vi "process_simple_analysis.vi"(8 "error in (no error)":errorcluster) -> (0 "error out":errorcluster)   [LabVIEW 2010]
uses:
  typedefs/control_analysis_enum.ctl
  typedefs/data_cluster.ctl
panel:
  out "Display sample rate":dbl caption="[Hz]"
  in  "Pixels to integrate":i32=1 min=1 max=1000 step=1
  in  "Display":enum32{"Raw data", "Integrated data"}(radio)
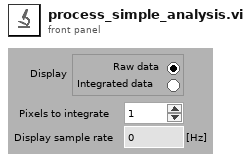
[diagram p1: front panel]
types:
  T1 = typedef "data_cluster.ctl" = cluster{"t0":dbl, "dt":dbl, "Channels":dbl[][]}
  T2 = typedef "control_analysis_enum.ctl" = enum16{"Init", "Analyze", "Reset", "Stop", "Quit"}
  T3 = cluster{"Control Analysis Enum":T2, "variant":variant}
  T4 = cluster{"Data_to_Display_Queue":refnum<queue>, "Data_to_Storage_Queue":refnum<queue>}
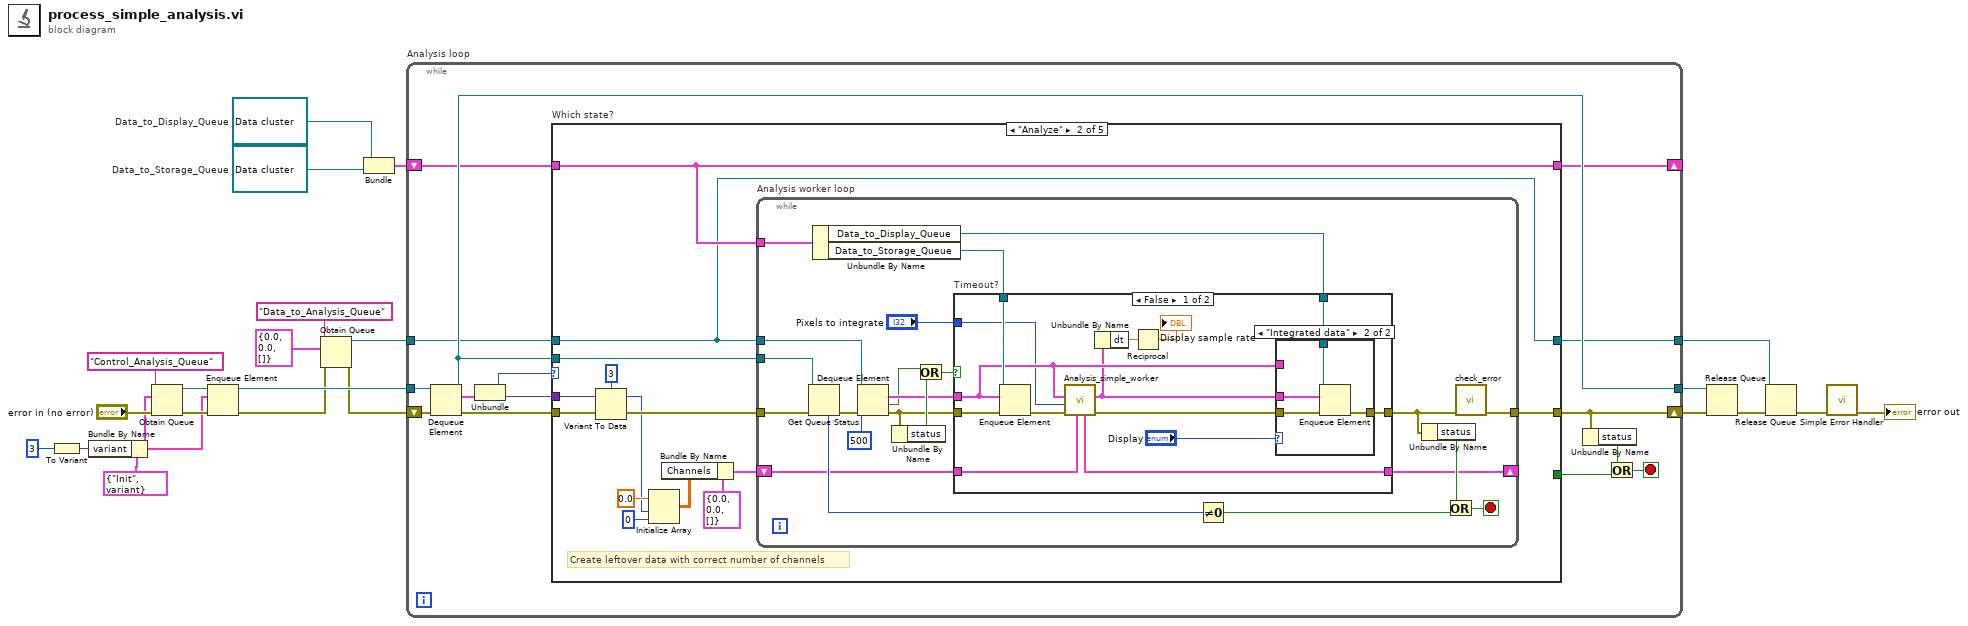
[diagram p0: block diagram]
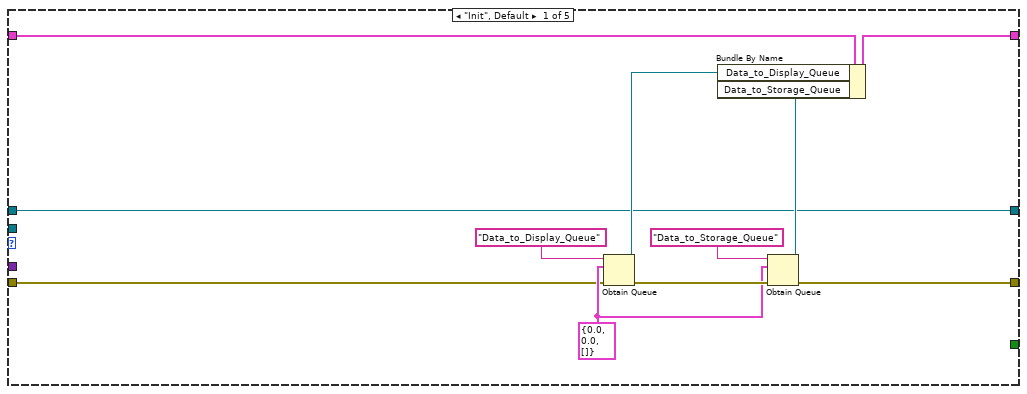
[diagram p2: hidden frame]
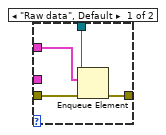
[diagram p3: hidden frame]
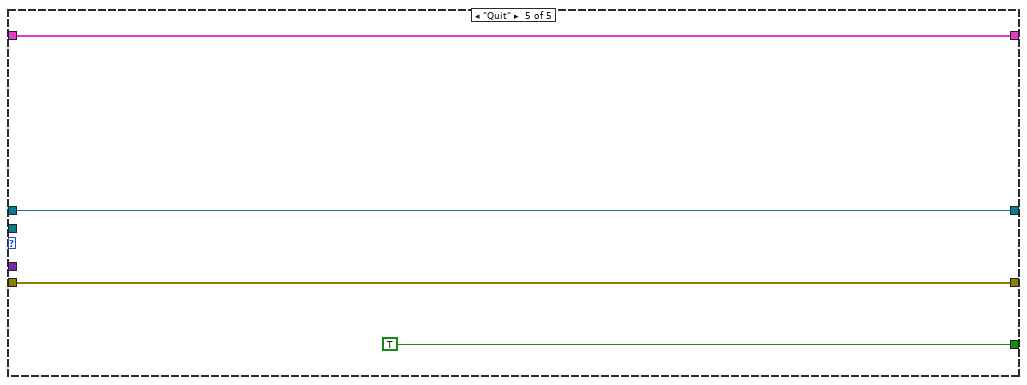
[diagram p7: hidden frame]
diagram:
  w7 = refnum<queue> refnum  # Data_to_Storage_Queue
  w8 = refnum<queue> refnum  # Data_to_Display_Queue
  n1 = To Variant(anything=3) -> (Variant=w2:variant)
  n2 = Bundle By Name(cluster=T3 {"Control Analysis Enum"=enum."Init", "variant"=variant}, "variant"=w2) -> (w1:T3)
  n3 = Obtain Queue(name (unnamed)="Control_Analysis_Queue", element data type=w1, error in (no error)="error in (no error)") -> (queue out=w20:refnum<queue>, error out=w21:errorcluster)  [unwired: 2 in, 1 out]
  n4 = Enqueue Element(queue=w20, element=w1, error in (no error)=w21) -> (queue out=w19:refnum<queue>, error out=w15:errorcluster)  [unwired: 1 in, 1 out]
  n5 = Obtain Queue(name (unnamed)="Data_to_Analysis_Queue", element data type=T1 {"t0"=0.0, "dt"=0.0, "Channels"=[]} ("Data cluster"), error in (no error)=w15) -> (queue out=w13:refnum<queue>, error out=w14:errorcluster)  [unwired: 2 in, 1 out]
  n6 = Bundle("Data_to_Display_Queue"=w8, "Data_to_Storage_Queue"=w7) -> (w12:T4)  [unwired: 1 in]
  n7 = while "Analysis loop" {
    shift-right: [w33] -> w18
    shift-left: w14 -> [w35]
    tunnel: w19 -> [w36]
    tunnel: [w28] -> w17
    tunnel: w13 -> [w24]
    shift-right: [w26] -> _
    shift-left: w12 -> [w27]
    tunnel: [w25] -> w10
    stop <- w37 stop-if-true
    n8 = Dequeue Element(queue=w36, error in (no error)=w35) -> (queue out=w28:refnum<queue>, element=w32:T3, error out=w34:errorcluster)  [unwired: 1 in, 1 out]
    n9 = Unbundle(w32) -> ("Control Analysis Enum"=w31:T2, "variant"=w30:variant)
    n10 = case "Which state?" shown="\"Analyze\"" w31 {
      tunnel: w34 -> [w39 w60 w110 w115 w119]
      tunnel: [w45 w63 w110 w115 w119] -> w33
      tunnel: w30 -> [_ w58 _ _ _]
      tunnel: [_ _ _ _ TRUE] -> w29
      tunnel: w28 -> [_ w62 _ _ _]
      tunnel: w27 -> [w48 w61 w112 w114 w117]
      tunnel: [w47 w61 w112 w114 w117] -> w26
      tunnel: [w41 w57 w111 w113 w116] -> w25
      tunnel: w24 -> [w41 w57 w111 w113 w116]
      frame "Init", Default {
        w40 = T1 {"t0"=0.0, "dt"=0.0, "Channels"=[]} ("Data cluster")
        n11 = Obtain Queue(name (unnamed)="Data_to_Display_Queue", element data type=w40, error in (no error)=w39) -> (queue out=w43:refnum<queue>, error out=w46:errorcluster)  [unwired: 2 in, 1 out]
        n12 = Obtain Queue(name (unnamed)="Data_to_Storage_Queue", element data type=w40, error in (no error)=w46) -> (queue out=w42:refnum<queue>, error out=w45:errorcluster)  [unwired: 2 in, 1 out]
        n13 = Bundle By Name(cluster=w48, "Data_to_Display_Queue"=w43, "Data_to_Storage_Queue"=w42) -> (w47:T4)
      }
      frame "Analyze" {
        # "Create leftover data with correct number of channels"
        n14 = Variant To Data(error in=w60, Variant=w58, type=3) -> (error out=w59:errorcluster, data=w50:i32)
        n15 = Initialize Array(0.0 ("element"), w50, 0 ("dimension size")) -> (w52:dbl[][])
        n16 = Bundle By Name(cluster=T1 {"t0"=0.0, "dt"=0.0, "Channels"=[]} ("Leftover data out"), "Channels"=w52) -> (w55:T1)
        n17 = while "Analysis worker loop" {
          tunnel: w59 -> [w84]
          tunnel: [w67] -> w63
          tunnel: w62 -> [w82]
          tunnel: w61 -> [w77]
          tunnel: w57 -> [w85]
          shift-right: [w73] -> _
          shift-left: w55 -> [w74]
          stop <- w78 stop-if-true
          n18 = Get Queue Status(queue=w82, error in (no error)=w84) -> (error out=w83:errorcluster, # elements in queue=w81:i32)  [unwired: 1 in, 6 out]
          n19 = Unbundle By Name(w77) -> ("Data_to_Display_Queue"=w75:refnum<queue>, "Data_to_Storage_Queue"=w76:refnum<queue>)
          n20 = Dequeue Element(queue=w85, timeout in ms (-1)=500, error in (no error)=w83) -> (element=w66:T1, timed out?=w65:bool, error out=w69:errorcluster)  [unwired: 1 out]
          n21 = Unbundle By Name(w69) -> ("status"=w71:bool)
          n22 = Or(x=w65, y=w71) -> (x .or. y?=w70:bool)
          n23 = case "Timeout?" shown="False" w70 {
            tunnel: [w99 w108] -> w68
            tunnel: w76 -> [w92 _]
            tunnel: w75 -> [w98 _]
            tunnel: w74 -> [w96 w109]
            tunnel: [w95 w109] -> w73
            tunnel: w69 -> [w94 w108]
            tunnel: w66 -> [w91 _]
            tunnel: "Pixels to integrate" -> [w89 _]
            frame False {
              n24 = Enqueue Element(queue=w92, element=w91, error in (no error)=w94) -> (error out=w93:errorcluster)  [unwired: 1 in, 2 out]
              n25 = call "Analysis_simple_worker.vi"("Leftover data in"=w96, "error in"=w93, "Pixels to integrate"=w89, "Data in"=w91) -> ("error out"=w90:errorcluster, "Data out"=w88:T1, "Leftover data out"=w95:T1)  [unwired: 3 in]
              n26 = Unbundle By Name(w88) -> ("dt"=w87:dbl)
              n27 = Reciprocal(x=w87) -> (1/x=→"Display sample rate":dbl)
              n28 = case shown="\"Integrated data\"" "Display" {
                tunnel: [w102 w107] -> w99
                tunnel: w98 -> [w101 w106]
                tunnel: w90 -> [w103 w105]
                tunnel: w91 -> [w100 _]
                tunnel: w88 -> [_ w104]
                frame "Raw data", Default {
                  n29 = Enqueue Element(queue=w101, element=w100, error in (no error)=w103) -> (error out=w102:errorcluster)  [unwired: 1 in, 2 out]
                }
                frame "Integrated data" {
                  n30 = Enqueue Element(queue=w106, element=w104, error in (no error)=w105) -> (error out=w107:errorcluster)  [unwired: 1 in, 2 out]
                }
              }
            }
            frame True {
            }
          }
          n31 = Not Equal To 0?(x=w81) -> (x != 0?=w80:bool)
          n32 = Unbundle By Name(w68) -> ("status"=w79:bool)
          n33 = Or(x=w79, y=w80) -> (x .or. y?=w78:bool)
          n34 = call "check_error.vi"("error in"=w68) -> ("error out"=w67:errorcluster)  [unwired: 10 in]
        }
      }
      frame "Reset" {
      }
      frame "Stop" {
      }
      frame "Quit" {
      }
    }
    n35 = Unbundle By Name(w33) -> ("status"=w38:bool)
    n36 = Or(x=w38, y=w29) -> (x .or. y?=w37:bool)
  }
  n37 = Release Queue(queue=w17, error in (no error)=w18) -> (error out=w11:errorcluster)  [unwired: 1 in, 2 out]
  n38 = Release Queue(queue=w10, error in (no error)=w11) -> (error out=w6:errorcluster)  [unwired: 1 in, 2 out]
  n39 = call <vilib>:"Simple Error Handler.vi"("error in (no error)"=w6) -> ("error out"=→"error out":errorcluster)  [unwired: 4 in, 4 out]
